vi "NIFPGA-MCS.start scan.vi"(0 "i ref in":refnum<vi>, 3 "ms timeout (10000)":i32=10000, 5 "error in (no error)":errorcluster) -> (14 "i ref out":refnum<vi>, 17 "timed out":bool, 19 "error out":errorcluster)   [LabVIEW 2014, in "NIFPGA-MCS.lvlib"]
doc: "Enables the hardware trigger and/or starts the acquisition."
uses:
  NIFPGA-MCS.lvlib
  CSCore/CSApplicationBaseClasses/DeviceBase/DeviceBase.lvlib
  CSinstr.lib/NI-FPGA-MCS/host/instrumentDriver/NI-FPGA-MCS_Driver.lvlib
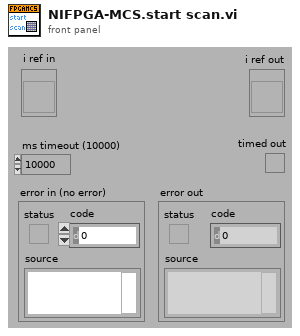
[diagram p1: front panel]
types:
  T1 = typedef "NIFPGA-MCS.lvlib/NIFPGA-MCS.i attribute.ctl" = cluster{"fpgaViRef":T2}
  T2 = typedef "NI-FPGA-MCS_Driver.lvlib/fpga_vi_ref.ctl" = refnum<k20>
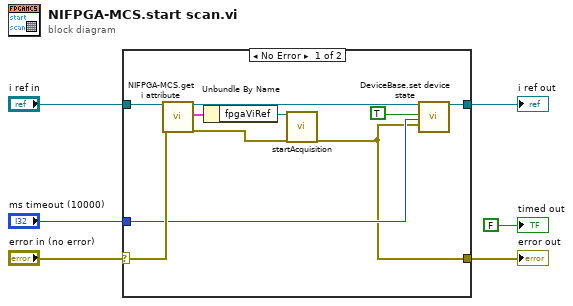
[diagram p0: block diagram]
diagram:
  n1 = case shown="No Error" "error in (no error)" {
    selector: "error in (no error)" -> [w15 w17]
    tunnel: "i ref in" -> [w16 w18]
    tunnel: [w12 w18] -> w4
    tunnel: [w7 w17] -> w3
    tunnel: "ms timeout (10000)" -> [w10 _]
    frame No Error {
      n2 = call "NIFPGA-MCS.get i attribute.vi"("i ref in"=w16, "error in (no error)"=w15) -> ("i ref out"=w8:refnum<vi>, "i attribute"=w13:T1, "error out"=w14:errorcluster)  [unwired: 15 in]
      n3 = Unbundle By Name(w13) -> ("fpgaViRef"=w11:T2)
      n4 = call "startAcquisition.vi"("fpga_vi_ref"=w11, "error in (no error)"=w14) -> ("error out"=w7:errorcluster)  [unwired: 16 in, 1 out]
      n5 = call "DeviceBase.set device state.vi"("i ref in"=w8, "implicit"=TRUE, "ms timeout (10000)"=w10, "device error"=w7) -> ("i ref out"=w12:refnum<vi>)  [unwired: 13 in, 2 out]
    }
    frame Error {
    }
  }
  "error out" <- w3
  "i ref out" <- w4
  "timed out" <- FALSE ("timed out")
